vi "Manual Build.vi"() -> ()   [LabVIEW 2019]
uses:
  <userlib>/LevyLab/Build Support/PostBuildSupport/PostBuildSupport.lvclass
panel:
  out "error out":errorcluster
  in  "Output Package File Path":path=path "E:/Github/Instrument Framework Tutorial/cypher-dashboard/build/package"
  in  "Product Name":string="Cypher Dashboard"
  in  "Package Version":string="0.1.0.1"
  in  "Package Source Folder":path=path "E:/Github/Instrument Framework Tutorial/cypher-dashboard/lvsrc"
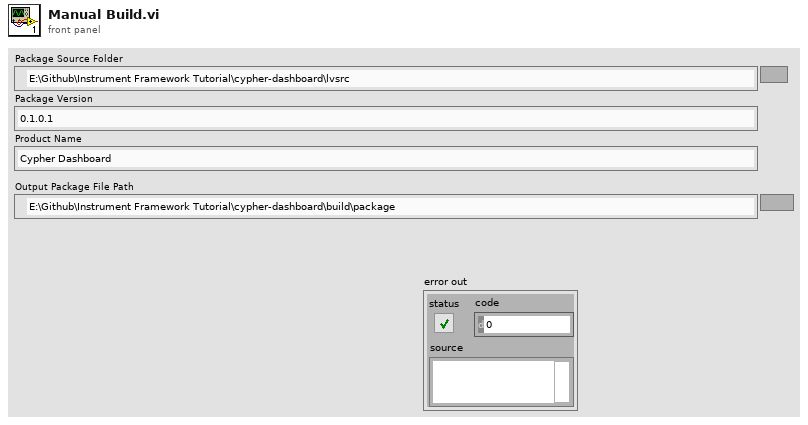
[diagram p1: front panel]
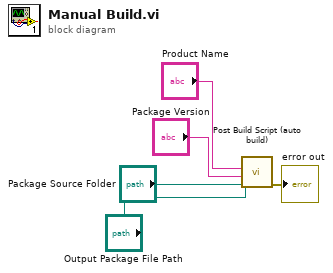
[diagram p0: block diagram]
diagram:
  n1 = call <userlib>:"Post Build Script (auto build).vi"("Package Source Folder"="Package Source Folder", "Package Version"="Package Version", "Product Name"="Product Name", "Output Package File Path"="Output Package File Path") -> ("error out"=→"error out":errorcluster)  [unwired: 7 in]
